vi "GetUsersDirectoryNames-subvi.vi"(0 "RAID root path":path, 1 "Error In":errorcluster) -> (2 "Username":string, 3 "directory names":string[](array[string]), 4 "Error Out":errorcluster)   [LabVIEW 2014]
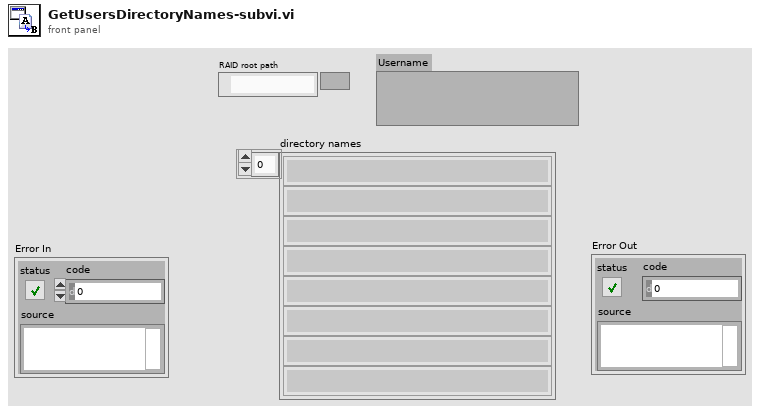
[diagram p1: front panel]
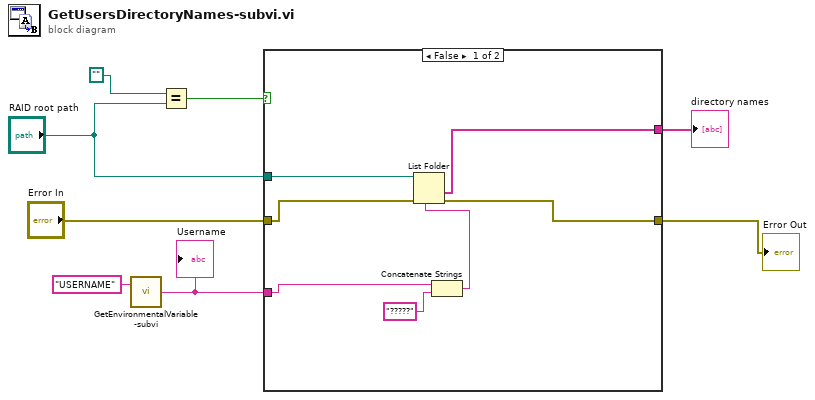
[diagram p0: block diagram]
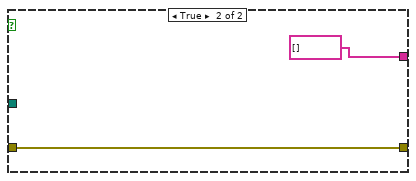
[diagram p2: hidden frame]
diagram:
  n1 = call "GetEnvironmentalVariable-subvi.vi"("Variable name"="USERNAME") -> ("Value"=w7:string)  [unwired: 1 in]
  "Username" <- w7
  n2 = Equal?(x=path "", y="RAID root path") -> (x = y?=w5:bool)
  n3 = case shown="False" w5 {
    tunnel: w7 -> [w12 _]
    tunnel: "Error In" -> [w15 w16]
    tunnel: [w9 string[] []] -> w3
    tunnel: [w10 w16] -> w1
    tunnel: "RAID root path" -> [w14 _]
    frame False {
      n4 = Concatenate Strings(w12, "?????" ("string")) -> (w11:string)
      n5 = List Folder(path=w14, pattern=w11, error in=w15) -> (folder names=w9:string[], error out=w10:errorcluster)  [unwired: 3 out]
    }
    frame True {
    }
  }
  "directory names" <- w3
  "Error Out" <- w1
